vi "dr_M_vertical.vi"(8 "error in":errorcluster, 10 "position":i32(slide) min=0 max=1200000 step=1000 scale=0.0..700000.0) -> (0 "error out":errorcluster)   [LabVIEW 2015, in "VIPM2.lvlib"]
doc: "<b>Vertical motor driver.</b>\ntype of movement: absolute.\nManages connection errors."
uses:
  VIPM2.lvlib
  <vilib>/Instr/_visa.llb/VISA Configure Serial Port (Instr).vi
panel:
  out "read answer":string
  out "Instruction sent":string
  # "Vertical motor driver"
  # "POS 280 000 for Na22\nPOS 668 700 for Co57\nPOS 200 000 for Ba133"
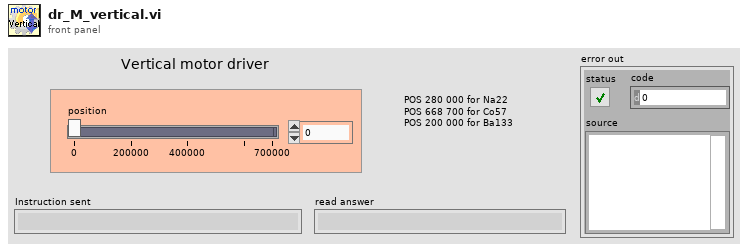
[diagram p1: front panel]
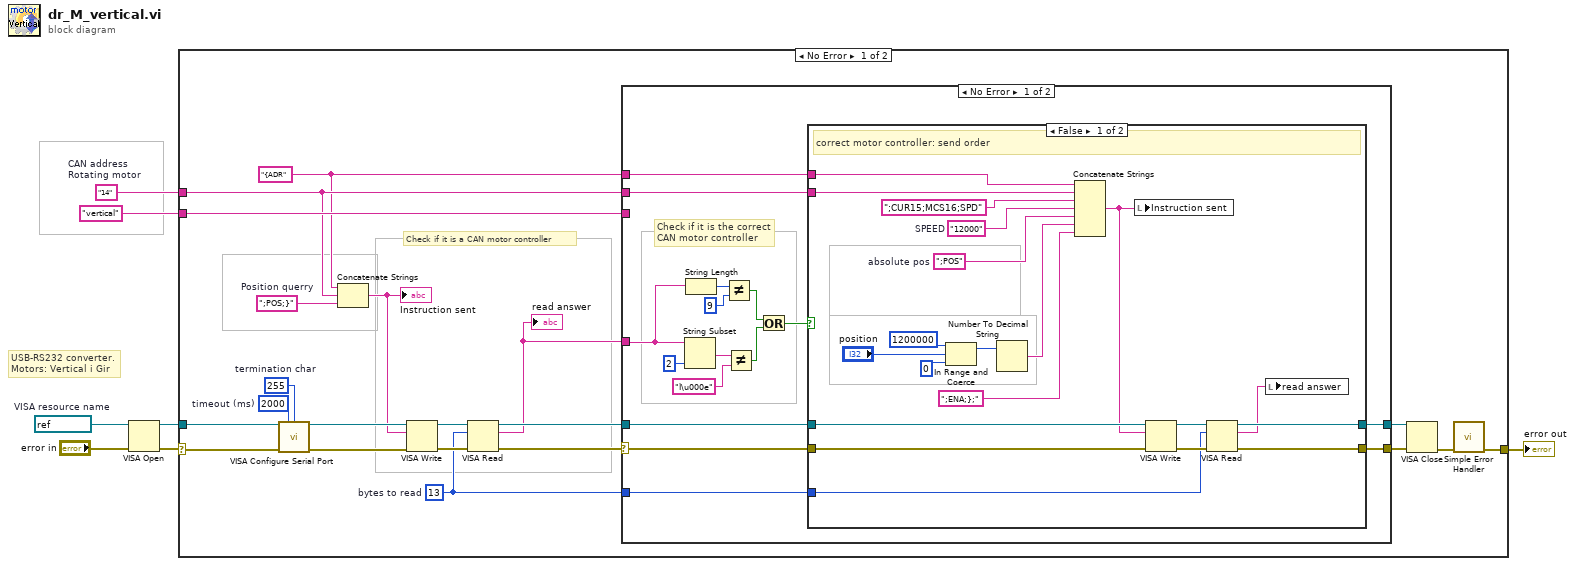
[diagram p0: block diagram]
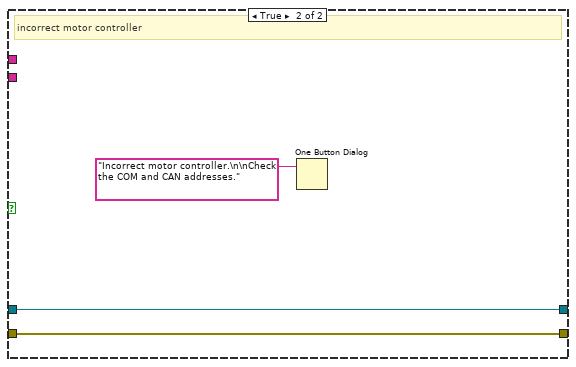
[diagram p2: hidden frame]
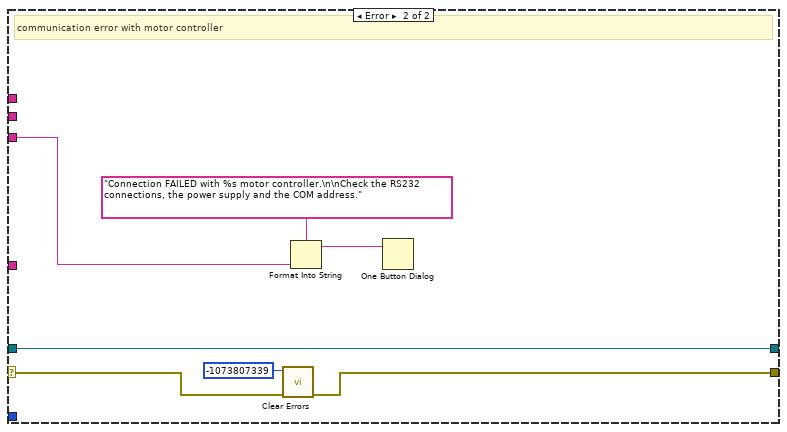
[diagram p3: hidden frame]
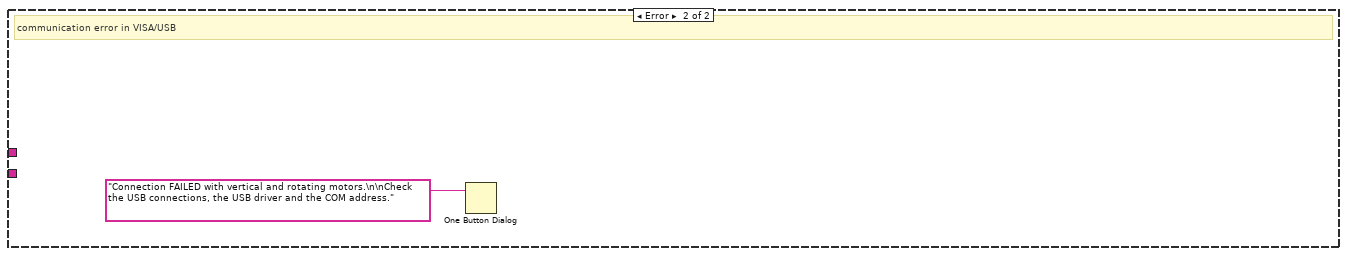
[diagram p4: hidden frame]
diagram:
  w4 = "14"  # CAN address Rotating motor
  w7 = refnum<visa-resource-name> "COM4"  # VISA resource name
  # "USB-RS232 converter.\nMotors: Vertical i Gir"
  n1 = VISA Open(error in (no error)="error in", VISA resource name=w7) -> (VISA resource name=w5:refnum<visa-resource-name>, error out=w6:errorcluster)  [unwired: 3 in]
  n2 = case shown="No Error" w6 {
    selector: w6 -> [w27 _]
    tunnel: w5 -> [w26 _]
    tunnel: w4 -> [w11 _]
    tunnel: "vertical" -> [w14 _]
    tunnel: [w8 _] -> w2
    frame No Error {
      w18 = u32 2000  # timeout (ms)
      w9 = u32 13  # bytes to read
      w24 = ";POS;}"  # Position querry
      w10 = "{ADR"
      w25 = u8 255  # termination char
      # "Check if it is a CAN motor controller"
      n3 = call-poly "VISA Configure Serial Port"("VISA resource name"=w26, "timeout (10sec)"=w18, "termination char\n(0xA = '\\n' = LF)"=w25, "error in (no error)"=w27) -> ("VISA resource name out"=w23:refnum<visa-resource-name>, "error out"=w22:errorcluster)  [unwired: 10 in]
      n4 = Concatenate Strings(w10, w11, w24) -> (w21:string)
      "Instruction sent" <- w21
      n5 = VISA Write(VISA resource name=w23, write buffer=w21, error in (no error)=w22) -> (VISA resource name out=w19:refnum<visa-resource-name>, error out=w20:errorcluster)  [unwired: 1 out]
      n6 = VISA Read(VISA resource name=w19, byte count=w9, error in (no error)=w20) -> (VISA resource name out=w16:refnum<visa-resource-name>, read buffer=w15:string, error out=w17:errorcluster)  [unwired: 1 out]
      "read answer" <- w15
      n7 = case shown="No Error" w17 {
        selector: w17 -> [w35 w69]
        tunnel: w16 -> [w34 w71]
        tunnel: w15 -> [w39 _]
        tunnel: w14 -> [_ w72]
        tunnel: [w33 w68] -> w13
        tunnel: [w32 w71] -> w12
        tunnel: w11 -> [w31 _]
        tunnel: w10 -> [w30 _]
        tunnel: w9 -> [w29 _]
        frame No Error {
          # "Check if it is the correct \nCAN motor controller"
          n8 = String Subset(string=w39, length (rest)=2 ("length (rest)")) -> (substring=w43:string)  [unwired: 1 in]
          n9 = String Length(string=w39) -> (length=w40:i32)
          n10 = Not Equal?(x=w40, y=9) -> (x != y?=w38:bool)
          n11 = Not Equal?(x=w43, y="Ì\u000e" ("substring")) -> (x != y?=w37:bool)
          n12 = Or(x=w38, y=w37) -> (x .or. y?=w36:bool)
          n13 = case shown="False" w36 {
            tunnel: w35 -> [w53 w67]
            tunnel: w34 -> [w54 w66]
            tunnel: [w56 w67] -> w33
            tunnel: [w52 w66] -> w32
            tunnel: w31 -> [w63 _]
            tunnel: w30 -> [w64 _]
            tunnel: w29 -> [w55 _]
            frame False {
              w49 = ";POS"  # absolute pos
              w61 = "12000"  # SPEED
              # "correct motor controller: send order"
              n14 = In Range and Coerce(upper limit=1200000, x="position", lower limit=0) -> (coerced(x)=w48:i32)  [unwired: 1 out]
              n15 = Number To Decimal String(number=w48) -> (decimal integer string=w59:string)  [unwired: 1 in]
              n16 = Concatenate Strings "Concatenate Strings"(w64, w63, ";CUR15;MCS16;SPD" ("string"), w61, w49, w59, ";ENA;};" ("string")) -> (w51:string)
              n17 = local write "Instruction sent"(w51) -> ()
              n18 = VISA Write(VISA resource name=w54, write buffer=w51, error in (no error)=w53) -> (VISA resource name out=w58:refnum<visa-resource-name>, error out=w57:errorcluster)  [unwired: 1 out]
              n19 = VISA Read(VISA resource name=w58, byte count=w55, error in (no error)=w57) -> (VISA resource name out=w52:refnum<visa-resource-name>, read buffer=w50:string, error out=w56:errorcluster)  [unwired: 1 out]
              n20 = local write "read answer"(w50) -> ()
            }
            frame True {
              # "incorrect motor controller"
              n21 = One Button Dialog(message="Incorrect motor controller.\n\nCheck the COM and CAN addresses.") -> ()  [unwired: 1 in, 1 out]
            }
          }
        }
        frame Error {
          # "communication error with motor controller"
          n22 = call <vilib>:"Clear Errors.vi"("error in (no error)"=w69, "specific error code to clear (0: all)"=-1073807339) -> ("error out"=w68:errorcluster)  [unwired: 4 in, 1 out]
          n23 = Format Into String "Format Into String"(format string="Connection FAILED with %s motor controller.\n\nCheck the RS232 connections, the power supply and the COM address." ("message"), w72) -> (resulting string=w73:string)  [unwired: 2 in, 1 out]
          n24 = One Button Dialog(message=w73) -> ()  [unwired: 1 in, 1 out]
        }
      }
      n25 = VISA Close(VISA resource name=w12, error in (no error)=w13) -> (error out=w28:errorcluster)
      n26 = call <vilib>:"Simple Error Handler.vi"("error in (no error)"=w28) -> ("error out"=w8:errorcluster)  [unwired: 4 in, 4 out]
    }
    frame Error {
      # "communication error in VISA/USB"
      n27 = One Button Dialog(message="Connection FAILED with vertical and rotating motors.\n\nCheck the USB connections, the USB driver and the COM address.") -> ()  [unwired: 1 in, 1 out]
    }
  }
  "error out" <- w2
